vi "mediaplaer-test.vi"() -> ()   [LabVIEW 2010]
uses:
  player_glo.vi
  playerlib.lvlib
panel:
  in  "balance":i8(slide) caption="Balance" scale=-10.0..10.0
  out "player referenz":refnum<vi>
  out "ende?":bool
  in  "schließen":bool
  in  "Status":ext(slide) scale=-1.0..251.354
  in  "File":path
  in  "stop":bool
  in  "pause":bool
  in  "play":bool
  in  "Volume":dbl(slide) scale=0.0..100.0
  # "supportet files: wav, snd, au, aif, aifc, aiff, wma, mp3, mid, midi, mi"
  # "Powered by"
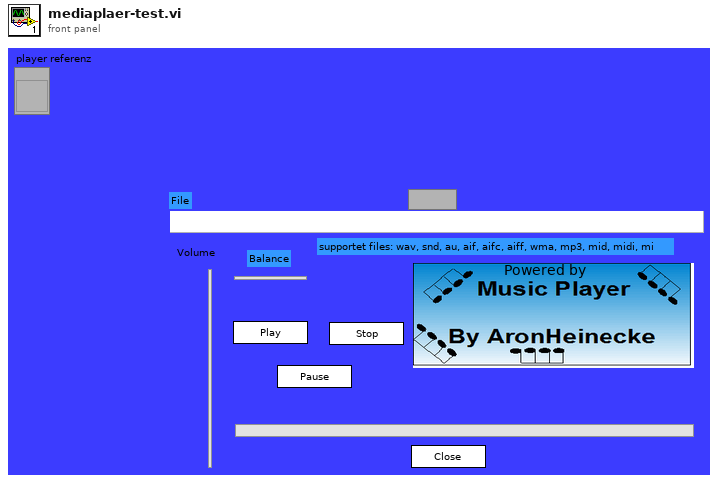
[diagram p1: front panel]
types:
  T1 = enum32{"Invalid", "Standard", "Closed", "Hidden", "Minimized", "Maximized"}
  T2 = enum32{"play and load URL", "stop", "pause", "default", "zeit insgesamt", "posotions änderung", "Titelinfo", "LoadURL(withoutplay)"}
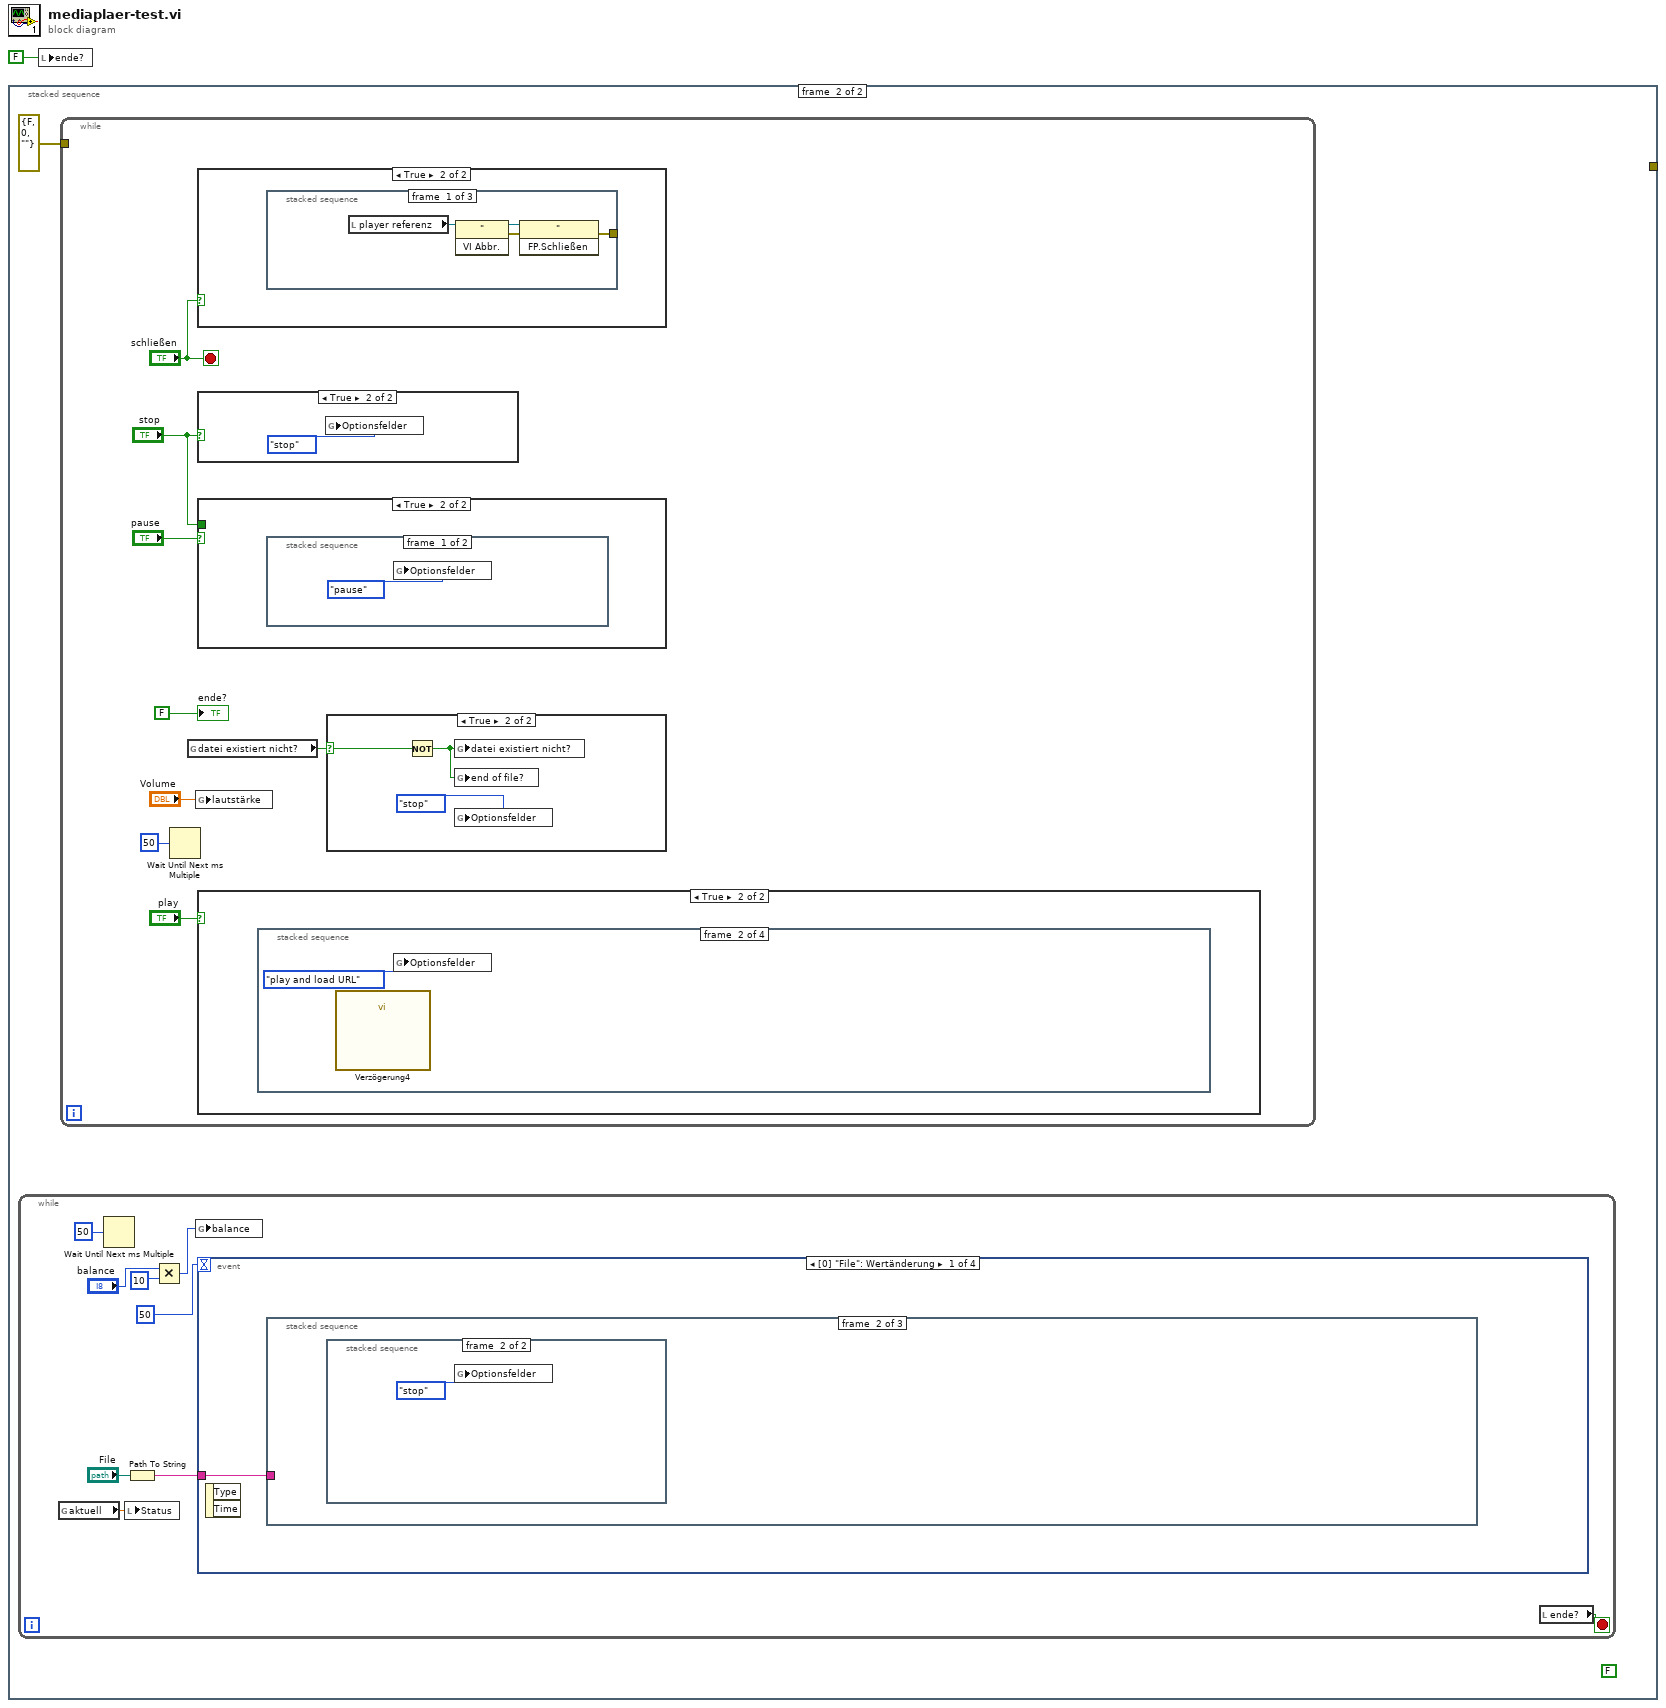
[diagram p0: block diagram]
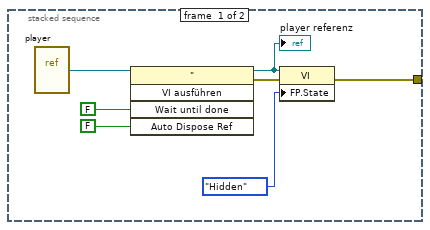
[diagram p2: hidden frame]
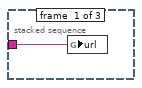
[diagram p3: hidden frame]
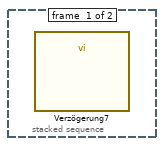
[diagram p4: hidden frame]
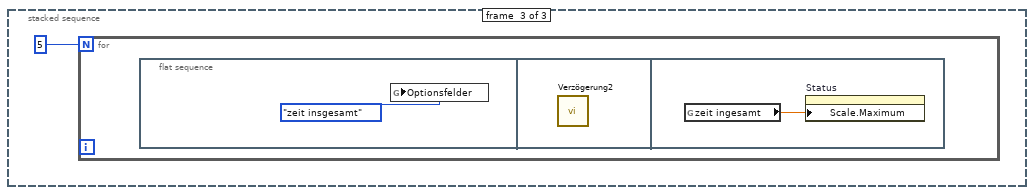
[diagram p5: hidden frame]
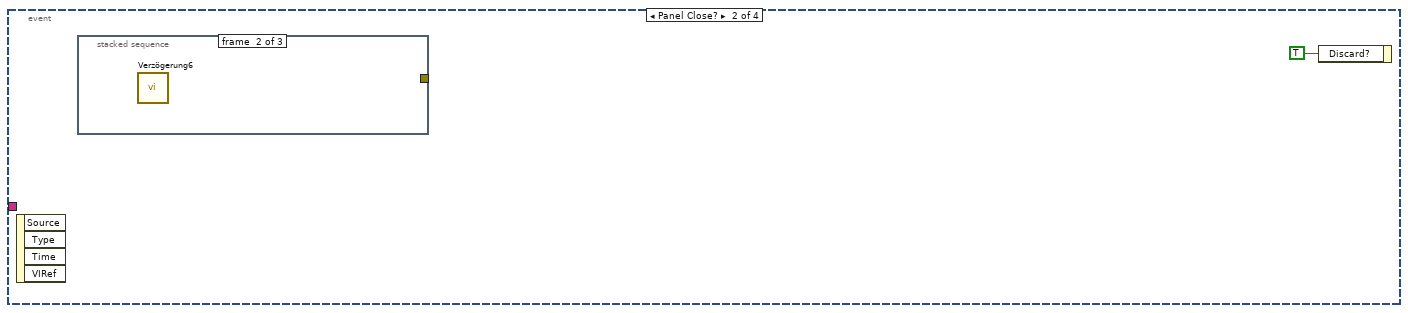
[diagram p6: hidden frame]
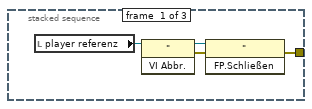
[diagram p7: hidden frame]
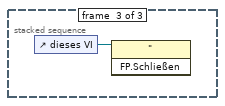
[diagram p8: hidden frame]
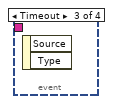
[diagram p9: hidden frame]
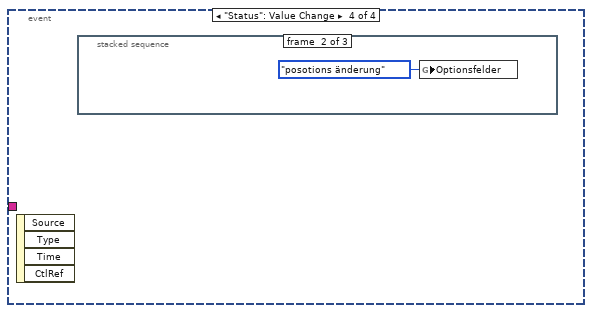
[diagram p10: hidden frame]
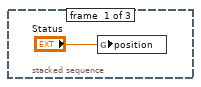
[diagram p11: hidden frame]
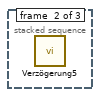
[diagram p15: hidden frame]
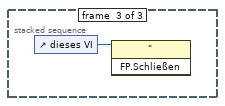
[diagram p16: hidden frame]
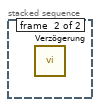
[diagram p18: hidden frame]
diagram:
  n1 = stacked-sequence {
    tunnel: [w3 _] -> _
    frame #0 {
      n2 = vi-ref "player.vi"() -> (w6:refnum<vi>)
      n3 = invoke class="\"" method="VI ausführen"(reference=w6, "Wait until done"=FALSE ("Warten bis beendet"), "Auto Dispose Ref"=FALSE ("Referenz automatisch schließen")) -> (reference out=w2:refnum<vi>, error out=w5:errorcluster)  [unwired: 2 in, 3 out]
      "player referenz" <- w2
      n4 = property class="VI"(reference=w2, error in=w5, "FP.State"=T1."Hidden" ("Frontpanel-Fenster:Status")) -> (error out=w3:errorcluster)  [unwired: 1 out]
    }
    frame #1 {
      (unwired) FALSE ("Neue Instanz öffnen (False)")
      n5 = while {
        stop <- w13 stop-if-true
        n6 = global read "player_glo.vi" "aktuell"() -> (w14:ext)
        n7 = Wait Until Next ms Multiple(millisecond multiple=u32 50 ("Vielfache von ms")) -> ()  [unwired: 1 out]
        n8 = local write "Status"(w14) -> ()
        n9 = Path To String(path="File") -> (string=w18:string)
        n10 = Multiply(x="balance", y=10) -> (x*y=w12:i32)
        n11 = global write "player_glo.vi" "balance"(w12) -> ()
        n12 = event shown="[0] \"File\": Wertänderung" {
          selector: _ -> [_ _ _ _]
          dyn-events: _ -> [_ _ _ _]
          timeout: 50 -> [_ _ _ _]
          tunnel: w18 -> [w19 _ _ _]
          event "File": Value Change {
            n13 = event-data() -> ()  [unwired: 3 out]
            n14 = stacked-sequence {
              tunnel: w19 -> [w20 _ _]
              frame #0 {
                n15 = global write "player_glo.vi" "url"(w20) -> ()
              }
              frame #1 {
                n16 = stacked-sequence {
                  frame #0 {
                    n17 = call "Verzögerung7"() -> ()  [unwired: 2 in, 10 out]
                  }
                  frame #1 {
                    n18 = global write "player_glo.vi" "Optionsfelder"(T2."stop" ("Optionsfelder")) -> ()
                  }
                }
              }
              frame #2 {
                n19 = for {
                  N: 5 -> [_]
                  n20 = flat-sequence {
                    frame #0 {
                      n21 = global write "player_glo.vi" "Optionsfelder"(T2."zeit insgesamt" ("Optionsfelder")) -> ()
                    }
                    frame #1 {
                      n22 = call "Verzögerung2"() -> ()  [unwired: 2 in, 10 out]
                    }
                    frame #2 {
                      n23 = global read "player_glo.vi" "zeit ingesamt"() -> (w24:ext)
                      n24 = property on="Status" class="Schieber (strikt)"("Scale.Maximum"=w24) -> ()  [unwired: 2 in, 2 out]
                    }
                  }
                }
              }
            }
          }
          event Panel Close? {
            n25 = event-data() -> ()  [unwired: 5 out]
            n26 = stacked-sequence {
              tunnel: [w26 _ _] -> _
              frame #0 {
                n27 = local read "player referenz"() -> (w29:refnum<vi>)
                n28 = invoke class="\"" method="VI Abbr."(reference=w29) -> (reference out=w28:refnum<vi>, error out=w27:errorcluster)  [unwired: 2 in, 1 out]
                n29 = invoke class="\"" method="FP.Schließen"(reference=w28, error in=w27) -> (error out=w26:errorcluster)  [unwired: 1 in, 2 out]
              }
              frame #1 {
                n30 = call "Verzögerung6"() -> ()  [unwired: 2 in, 10 out]
              }
              frame #2 {
                n31 = control-ref of="dieses VI"() -> (w30:refnum<vi>)
                n32 = invoke class="\"" method="FP.Schließen"(reference=w30) -> ()  [unwired: 2 in, 3 out]
              }
            }
            n33 = event-data("Discard?"=TRUE ("Verwerfen?")) -> ()  [unwired: 1 in, 1 out]
          }
          event Timeout {
            n34 = event-data() -> ()  [unwired: 3 out]
          }
          event "Status": Value Change {
            n35 = event-data() -> ()  [unwired: 5 out]
            n36 = stacked-sequence {
              frame #0 {
                n37 = global write "player_glo.vi" "position"("Status") -> ()
              }
              frame #1 {
                n38 = global write "player_glo.vi" "Optionsfelder"(T2."posotions änderung" ("Optionsfelder")) -> ()
              }
              frame #2 {
              }
            }
          }
        }
        n39 = local read "ende?"() -> (w13:bool)
      }
      n40 = while {
        tunnel: errorcluster {"status"=FALSE, "code"=0, "source"=""} ("error out") -> [_]
        stop <- "schließen" stop-if-true
        n41 = Wait Until Next ms Multiple(millisecond multiple=u32 50 ("Vielfache von ms")) -> ()  [unwired: 1 out]
        n42 = global read "player_glo.vi" "datei existiert nicht?"() -> (w33:bool)
        n43 = global write "player_glo.vi" "lautstärke"("Volume") -> ()
        n44 = case shown="True" "schließen" {
          frame False {
          }
          frame True {
            n45 = stacked-sequence {
              tunnel: [w44 _ _] -> _
              frame #0 {
                n46 = local read "player referenz"() -> (w47:refnum<vi>)
                n47 = invoke class="\"" method="VI Abbr."(reference=w47) -> (reference out=w46:refnum<vi>, error out=w45:errorcluster)  [unwired: 2 in, 1 out]
                n48 = invoke class="\"" method="FP.Schließen"(reference=w46, error in=w45) -> (error out=w44:errorcluster)  [unwired: 1 in, 2 out]
              }
              frame #1 {
                n49 = call "Verzögerung5"() -> ()  [unwired: 2 in, 10 out]
              }
              frame #2 {
                n50 = control-ref of="dieses VI"() -> (w48:refnum<vi>)
                n51 = invoke class="\"" method="FP.Schließen"(reference=w48) -> ()  [unwired: 2 in, 3 out]
              }
            }
          }
        }
        n52 = case shown="True" "stop" {
          frame False {
          }
          frame True {
            n53 = global write "player_glo.vi" "Optionsfelder"(T2."stop" ("Optionsfelder")) -> ()
          }
        }
        n54 = case shown="True" "pause" {
          tunnel: "stop" -> [_ _]
          frame False {
          }
          frame True {
            n55 = stacked-sequence {
              frame #0 {
                n56 = global write "player_glo.vi" "Optionsfelder"(T2."pause" ("Optionsfelder")) -> ()
              }
              frame #1 {
                n57 = call "Verzögerung"() -> ()  [unwired: 2 in, 10 out]
              }
            }
          }
        }
        n58 = case shown="True" "play" {
          frame False {
          }
          frame True {
            n59 = stacked-sequence {
              frame #0 {
                n60 = local read "File"() -> (w52:path)
                n61 = Path To String(path=w52) -> (string=w51:string)
                n62 = global write "player_glo.vi" "url"(w51) -> ()
              }
              frame #1 {
                n63 = call "Verzögerung4"() -> ()  [unwired: 2 in, 10 out]
                n64 = global write "player_glo.vi" "Optionsfelder"(T2."play and load URL" ("Optionsfelder")) -> ()
              }
              frame #2 {
                n65 = stacked-sequence {
                  frame #0 {
                    n66 = global write "player_glo.vi" "position"(0.0 ("position")) -> ()
                  }
                  frame #1 {
                    n67 = global write "player_glo.vi" "Optionsfelder"(T2."posotions änderung" ("Optionsfelder")) -> ()
                  }
                }
              }
              frame #3 {
                n68 = flat-sequence {
                  frame #0 {
                    n69 = global write "player_glo.vi" "Optionsfelder"(T2."zeit insgesamt" ("Optionsfelder")) -> ()
                  }
                  frame #1 {
                    n70 = call "Verzögerung3"() -> ()  [unwired: 2 in, 10 out]
                  }
                  frame #2 {
                    n71 = global read "player_glo.vi" "zeit ingesamt"() -> (w57:ext)
                    n72 = property on="Status" class="Schieber (strikt)"("Scale.Maximum"=w57) -> ()  [unwired: 2 in, 2 out]
                  }
                }
              }
            }
          }
        }
        n73 = case shown="True" w33 {
          selector: w33 -> [_ w43]
          frame False {
          }
          frame True {
            n74 = Not(x=w43) -> (.not. x?=w42:bool)
            n75 = global write "player_glo.vi" "datei existiert nicht?"(w42) -> ()
            n76 = global write "player_glo.vi" "end of file?"(w42) -> ()
            n77 = global write "player_glo.vi" "Optionsfelder"(T2."stop" ("Optionsfelder")) -> ()
          }
        }
        "ende?" <- FALSE ("ende?")
      }
    }
  }
  n78 = local write "ende?"(FALSE ("ende?")) -> ()
